vi "cdaq_blinky.vi"   [LabVIEW 2023]
uses:
  <vilib>/NI_Real-Time Target Support.lvlib
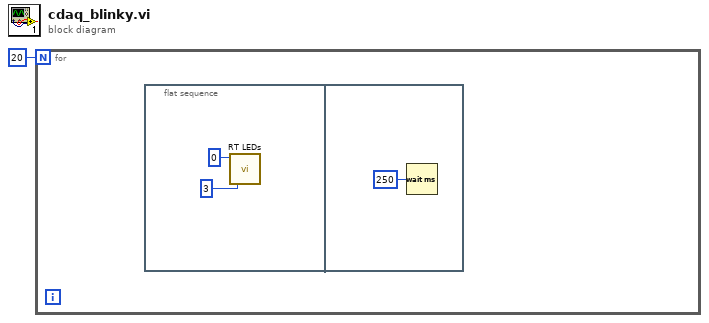
[diagram p0: block diagram]
diagram:
  n1 = for {
    N: 20 -> [_]
    n2 = flat-sequence {
      frame #0 {
        n3 = call <vilib>:"RT LEDs.vi"("State"=3, "LED Num"=0) -> ()  [unwired: 4 in, 2 out]
      }
      frame #1 {
        n4 = Wait (ms)(milliseconds to wait=u32 250) -> ()  [unwired: 1 out]
      }
    }
  }
